vi "demo1_sub1.vi"(8 "error in (no error)":errorcluster, 11 "VI Reference In":refnum<vi>) -> (0 "error out":errorcluster, 3 "VI Reference Out":refnum<vi>)   [LabVIEW 2016]
uses:
  main/apis/Stimulus/ValueSignalByPathString.vi
  <vilib>/addons/_JKI Toolkits/Caraya/classes/Test/Test.lvclass
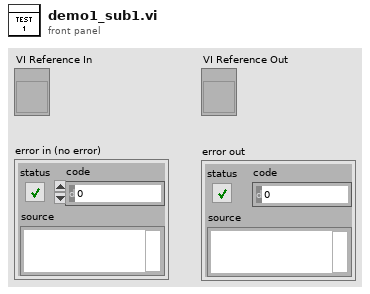
[diagram p1: front panel]
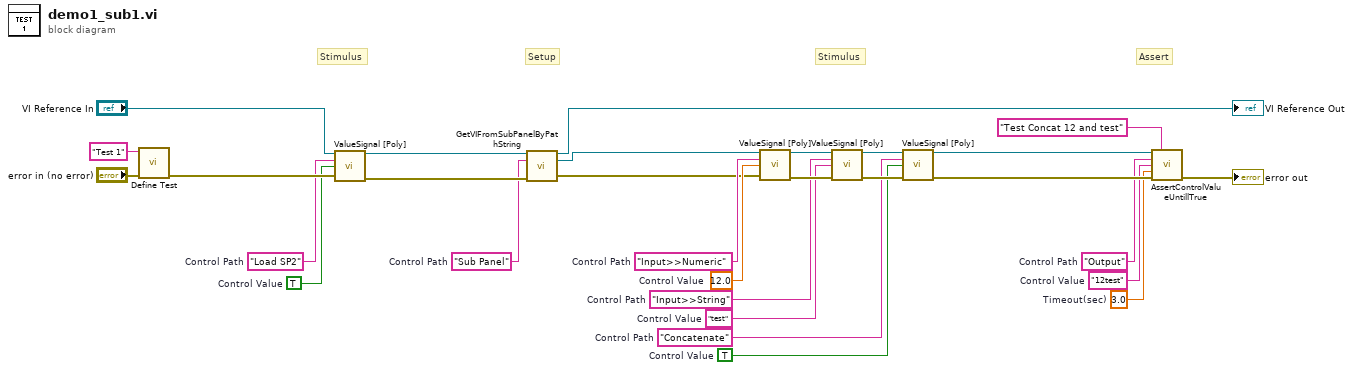
[diagram p0: block diagram]
diagram:
  w4 = "Input>>String"  # Control Path
  w5 = "Sub Panel"  # Control Path
  w10 = 3.0  # Timeout(sec)
  w12 = "12test"  # Control Value
  w13 = "Output"  # Control Path
  w16 = "Input>>Numeric"  # Control Path
  w17 = TRUE  # Control Value
  w18 = "Concatenate"  # Control Path
  w21 = "test"  # Control Value
  w24 = 12.0  # Control Value
  w25 = TRUE  # Control Value
  w26 = "Load SP2"  # Control Path
  # "Assert"
  # "Setup"
  # "Stimulus"
  # "Stimulus"
  n1 = call <vilib>:"Define Test.vi"("error in (no error)"="error in (no error)", "Label (VI Title)"="Test 1") -> ("error out"=w28:errorcluster)  [unwired: 9 in]
  n2 = call-poly "ValueSignal [Poly].vi"("VI Reference In"="VI Reference In", "Control Name"=w26, "Value (Signaling)"=w25, "error in"=w28) -> ("VI Reference Out"=w8:refnum<vi>, "error out"=w9:errorcluster)  [unwired: 10 in]
  n3 = call "GetVIFromSubPanelByPathString.vi"("VI Reference In"=w8, "SubPanel Path"=w5, "error in"=w9) -> ("VI Reference Out"=→"VI Reference Out":refnum<vi>, "SubPanel VI Reference"=w6:refnum<vi>, "error out"=w7:errorcluster)  [unwired: 10 in]
  n4 = call-poly "ValueSignal [Poly].vi"("VI Reference In"=w6, "Control Name"=w16, "Value (Signaling)"=w24, "error in"=w7) -> ("VI Reference Out"=w22:refnum<vi>, "error out"=w23:errorcluster)  [unwired: 10 in]
  n5 = call-poly "ValueSignal [Poly].vi"("VI Reference In"=w22, "Control Name"=w4, "Value (Signaling)"=w21, "error in"=w23) -> ("VI Reference Out"=w19:refnum<vi>, "error out"=w20:errorcluster)  [unwired: 10 in]
  n6 = call-poly "ValueSignal [Poly].vi"("VI Reference In"=w19, "Control Name"=w18, "Value (Signaling)"=w17, "error in"=w20) -> ("VI Reference Out"=w14:refnum<vi>, "error out"=w15:errorcluster)  [unwired: 10 in]
  n7 = call "AssertControlValueUntillTrue.vi"("VI Reference In"=w14, "Label"="Test Concat 12 and test", "Control Name"=w13, "Control Value"=w12, "Timeout(5 sec)"=w10, "error out"=w15) -> ("error out 2"=→"error out":errorcluster)  [unwired: 8 in, 1 out]
